vi "unlock.vi"(7 "Unlock?":bool, 8 "error in (no error)":errorcluster, 11 "Client in":refnum<class "Client.lvclass">) -> (0 "error out":errorcluster, 3 "Client out":refnum<class "Client.lvclass">)   [LabVIEW 2013, in "MQTT Client.lvlib" / "Client.lvclass"]
uses:
  Client.lvclass
  Client.lvclass/Client.ctl
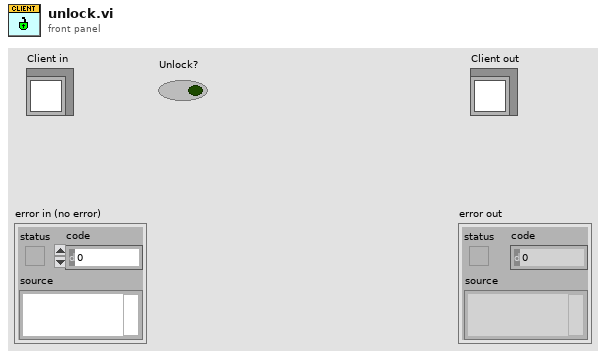
[diagram p1: front panel]
types:
  T1 = typedef "Semaphore RefNum" = refnum<k1>
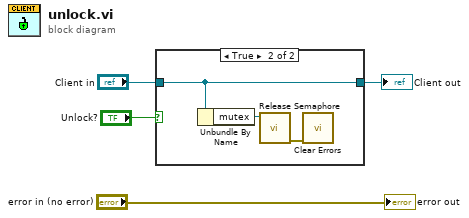
[diagram p0: block diagram]
diagram:
  n1 = case shown="True" "Unlock?" {
    tunnel: "Client in" -> [w5 w6]
    tunnel: [w5 w6] -> w2
    frame False {
    }
    frame True {
      n2 = Unbundle By Name(w6) -> ("mutex"=w7:T1)
      n3 = call <vilib>:"Release Semaphore.vi"("semaphore"=w7) -> ("error out"=w8:errorcluster)  [unwired: 5 in, 1 out]
      n4 = call <vilib>:"Clear Errors.vi"("error in (no error)"=w8) -> ()  [unwired: 6 in, 1 out]
    }
  }
  "Client out" <- w2
  "error out" <- "error in (no error)"
